vi "2's Comp To Signed Double.vi"(1 "2's ccomp":dbl) -> (0 "Signed Double":dbl)   [LabVIEW 2020]
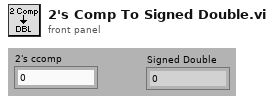
[diagram p1: front panel]
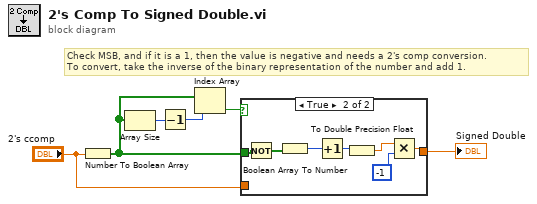
[diagram p0: block diagram]
diagram:
  # "Check MSB, and if it is a 1, then the value is negative and needs a 2's comp conversion.\nTo convert, take the inverse of the binary representation of the number and add 1."
  n1 = Number To Boolean Array(number="2's ccomp") -> (Boolean array=w1:bool[])
  n2 = Array Size(array=w1) -> (size(s)=w5:i32)
  n3 = Decrement(x=w5) -> (x-1=w4:i32)
  n4 = Index Array(array=w1, index=w4) -> (element=w3:bool)
  n5 = case shown="True" w3 {
    tunnel: [w7 w12] -> w6
    tunnel: w1 -> [_ w8]
    tunnel: "2's ccomp" -> [w7 _]
    frame False {
    }
    frame True {
      n6 = Not(x=w8) -> (.not. x?=w14:bool[])
      n7 = Boolean Array To Number(Boolean array=w14) -> (number=w13:u32)
      n8 = Increment(x=w13) -> (x+1=w10:u32)
      n9 = To Double Precision Float(number=w10) -> (double precision float=w9:dbl)
      n10 = Multiply(x=w9, y=-1) -> (x*y=w12:dbl)
    }
  }
  "Signed Double" <- w6
